vi "Pre Launch Init.vi"(11 "Nested in":refnum<class "User Interface.lvclass">) -> (0 "error out":errorcluster, 3 "Nested out":refnum<class "User Interface.lvclass">)   [LabVIEW 2020, in "User Interface.lvlib" / "User Interface.lvclass"]
doc: "(<B>Filename</B>: Actor Framework.lvlib:Actor.lvclass:Pre Launch Init.vi)\n\nDefines behavior that occurs after the Launch Nested Actor method is invoked but before the actor's Actor Core method begins running.\n\nBy default, this method does nothing. A descendant class may override it to define behavior."
uses:
  User Interface.lvclass
  User Interface.lvclass/User Interface.ctl
  <vilib>/ActorFramework/Actor/Actor.lvclass
  User Interface Messages/Update Status Msg/Update Status Msg.lvclass
  C:/Program Files (x86)/National Instruments/LabVIEW 2020/vi.lib/ActorFramework/Actor/Actor.lvclass
  D:/Storage/Source Code/Clase AF/ClaseAF/08 Acquisition AF/User Interface/User Interface.lvclass
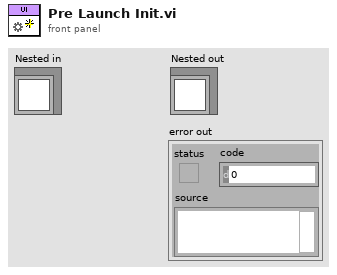
[diagram p1: front panel]
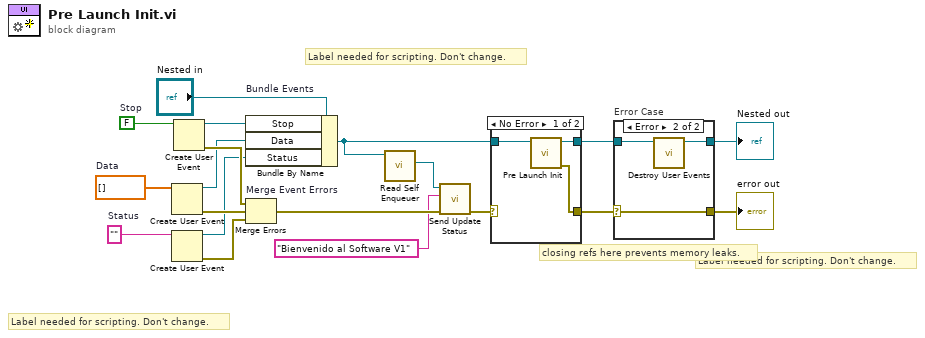
[diagram p0: block diagram]
diagram:
  w8 = ""  # Status
  w11 = dbl[] []  # Data
  w18 = FALSE  # Stop
  # "Label needed for scripting. Don't change."
  # "Label needed for scripting. Don't change."
  # "Label needed for scripting. Don't change."
  # "closing refs here prevents memory leaks."
  n1 = Create User Event(user event datatype=w11) -> (user event=w10:refnum<user-event>, error out=w9:errorcluster)  [unwired: 1 in]
  n2 = Create User Event(user event datatype=w8) -> (user event=w7:refnum<user-event>, error out=w6:errorcluster)  [unwired: 1 in]
  n3 = Create User Event(user event datatype=w18) -> (user event=w15:refnum<user-event>, error out=w17:errorcluster)  [unwired: 1 in]
  n4 = Bundle By Name "Bundle Events"(cluster="Nested in", "Stop"=w15, "Data"=w10, "Status"=w7) -> (w5:refnum<class "User Interface.lvclass">)
  n5 = Merge Errors "Merge Event Errors"(w17, w9, w6) -> (w4:errorcluster)
  n6 = call <vilib>:"Read Self Enqueuer.vi"("Actor"=w5) -> ("Self Enqueuer"=w2:refnum<class "Message Enqueuer.lvclass">)  [unwired: 10 in]
  n7 = call "Send Update Status.vi"("error in (no error)"=w4, "Status"="Bienvenido al Software V1", "Message Enqueuer"=w2) -> ("error out"=w3:errorcluster)  [unwired: 7 in, 1 out]
  n8 = case shown="No Error" w3 {
    selector: w3 -> [_ w24]
    tunnel: [w22 w23] -> w13
    tunnel: w5 -> [w21 w23]
    tunnel: [w20 w24] -> w12
    frame No Error {
      n9 = call-parent "Pre Launch Init.vi"("Actor in"=w21) -> ("error out"=w20:errorcluster, "Actor out"=w22:refnum<class "User Interface.lvclass">)  [unwired: 9 in]
    }
    frame Error {
    }
  }
  n10 = case "Error Case" shown="Error" w12 {
    selector: w12 -> [w25 w29]
    tunnel: w13 -> [w26 w28]
    tunnel: [w26 w27] -> w16
    tunnel: [w25 w29] -> w14
    frame No Error {
    }
    frame Error {
      n11 = call "Destroy User Events.vi"("UI Template in"=w28) -> ("UI Template out"=w27:refnum<class "User Interface.lvclass">)  [unwired: 10 in]
    }
  }
  "error out" <- w14
  "Nested out" <- w16
